vi "Code 0.0.4.vi"(8 "error in (no error)":errorcluster, 9 "Drv":u8(ring) items=["Drv 1", "Drv 2"], 10 "Port":u16=8030) -> (0 "error out":errorcluster)   [LabVIEW 2017]
panel:
  out "Array 2":u8[][](array[numeric])
  out "Array":u16[](array[numeric])
  in  "x":bool
  out "array":i32[][](array[numeric])
  out "O":i32[](array[numeric])
  out "Data1Send":bool
  out "DataBSend":bool
  out "Array 5":u16[](array[numeric]) format="%.0x"
  out "Array 4":u16[](array[numeric]) format="%.0x"
  out "Numeric":i32
  out "CheckSumData2":u16 format="%.0x"
  in  "DataBSendFlag":bool
  out "CheckSumData1":u16 format="%.0x"
  in  "Data1SendFlag":bool
  in  "HeaderFlag":bool
  out "(hi.lo) 3":u16 format="%.0x"
  out "(hi.lo) 2":u16 format="%.0x"
  out "Drv Out":u8[](array[numeric]) format="%.0x"
  out "E1b":u8 format="%.0x"
  in  "CatchNetworkFlag":bool
  out "E1a":u8 format="%.0x"
  out "State":i32
  in  "stop Listen":bool
  in  "status":bool
  out "conn ID":refnum<k5>
  out "Error List":string
  in  "Next Button":bool
  in  "File Path Control":path
  out "Status":bool
  out "cmd Sent":bool
  out "CheckSumArray":u16[][](array[numeric]) format="%.0x"
  out "CheckSum":bool[][](array[boolean])
  out "CheckSum DataB":u16 format="%.0x"
  out "CheckSum Data":u16 format="%.0x"
  out "Array 3":u16[][](array[numeric]) format="%.0x"
  out "Num of Data packet":i32
  out "Writting Data":bool
  out "Size of Text File":i32
  out "Full Text File":u8[](array[numeric]) format="%.0x"
  out "All bytes in file in HEX U8":u8[](array[numeric]) format="%02x"
  out "Send Header":bool
  out "AutoBaud Success":bool
  out "sumHeader":u16 format="%.0x"
  in  "AutoBaudFalg":bool
  # "Ver 0.0.4"
  # "Header"
  # "AA08 0000 0000 0000 0000 0000 0000 0000 0000 3E00 8DE6"
  # "Boot\n495D 4100 0001 0000 0050 F8"
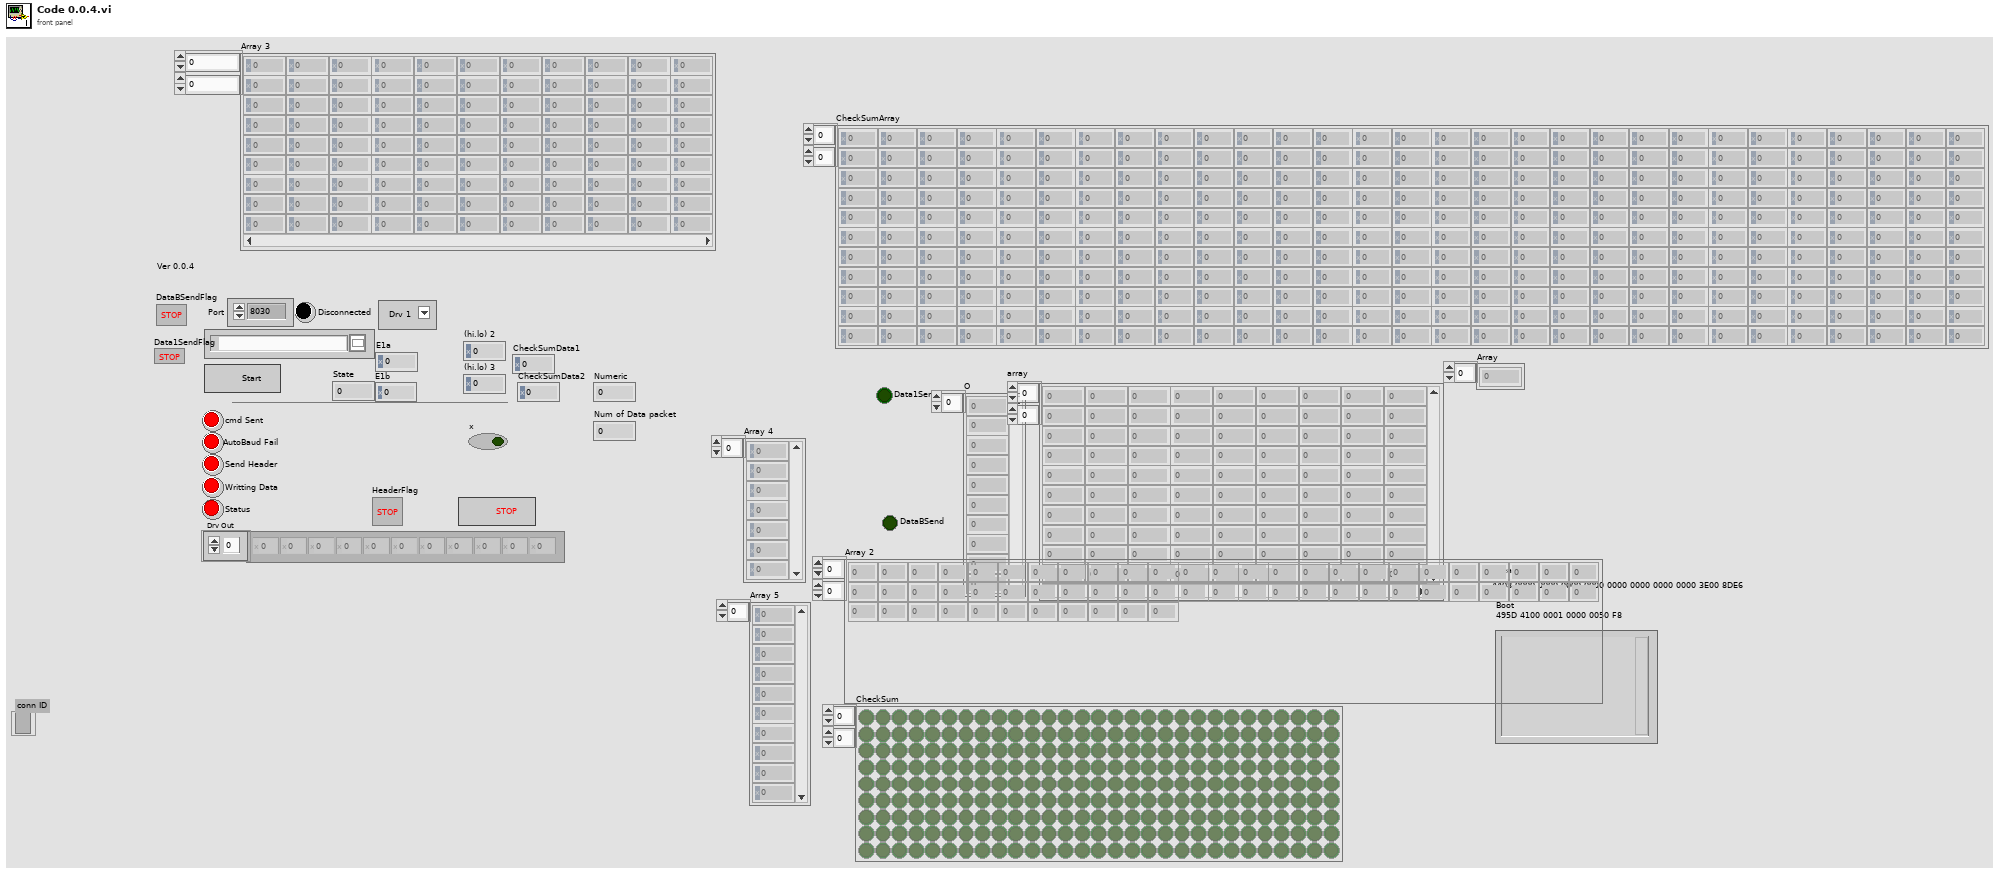
[diagram p1: front panel]
types:
  T1 = enum16{"open", "replace", "create", "open or create", "replace or create", "replace or create with confirmation"}
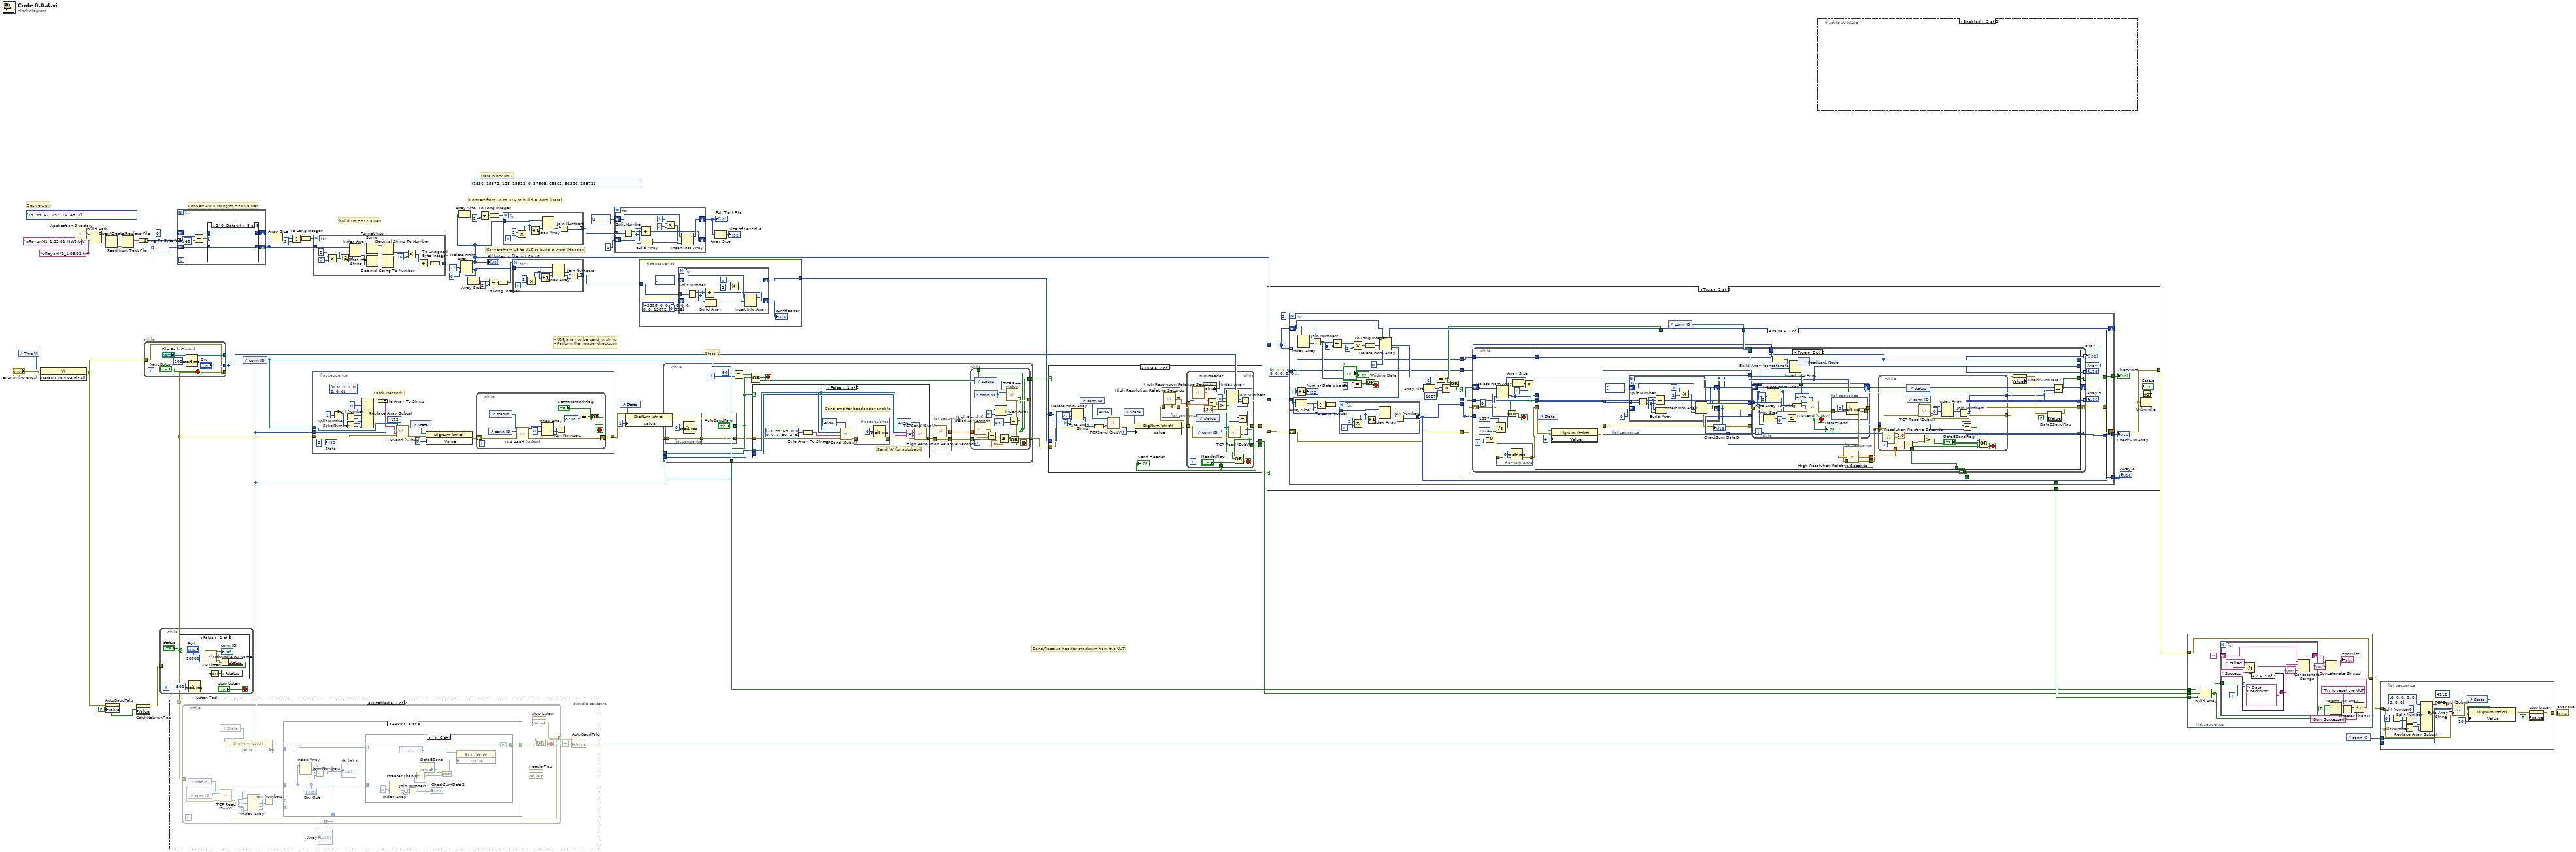
[diagram p0: block diagram]
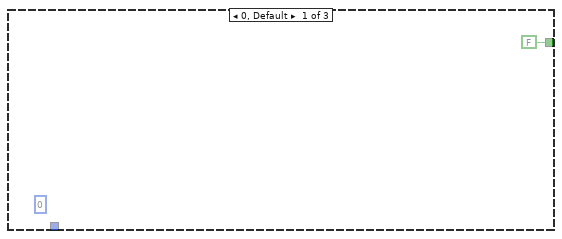
[diagram p2: hidden frame]
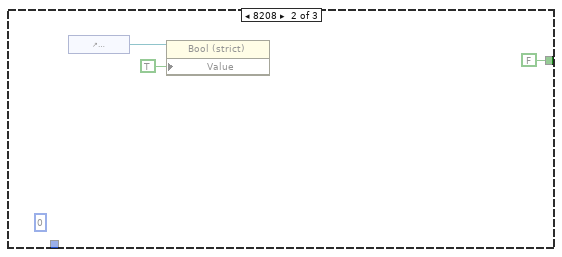
[diagram p3: hidden frame]
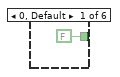
[diagram p4: hidden frame]
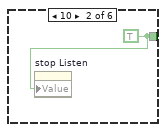
[diagram p5: hidden frame]
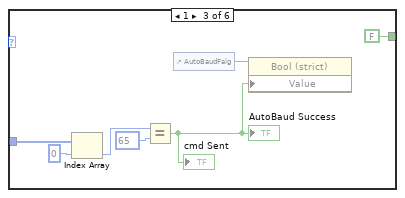
[diagram p6: hidden frame]
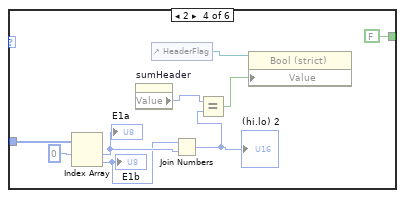
[diagram p7: hidden frame]
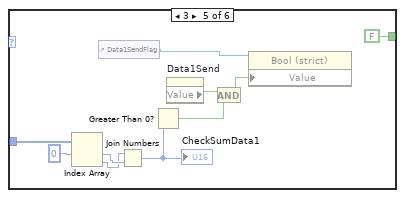
[diagram p8: hidden frame]
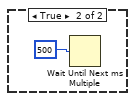
[diagram p11: hidden frame]
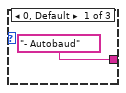
[diagram p12: hidden frame]
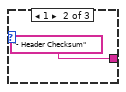
[diagram p13: hidden frame]
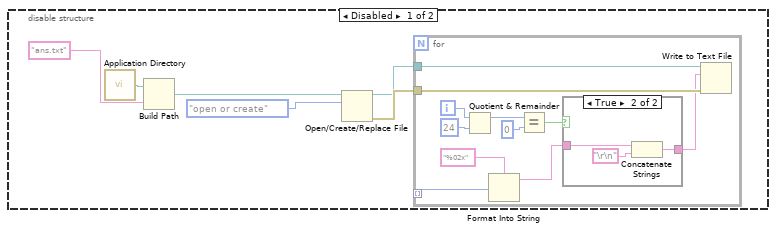
[diagram p14: hidden frame]
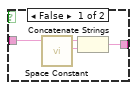
[diagram p15: hidden frame]
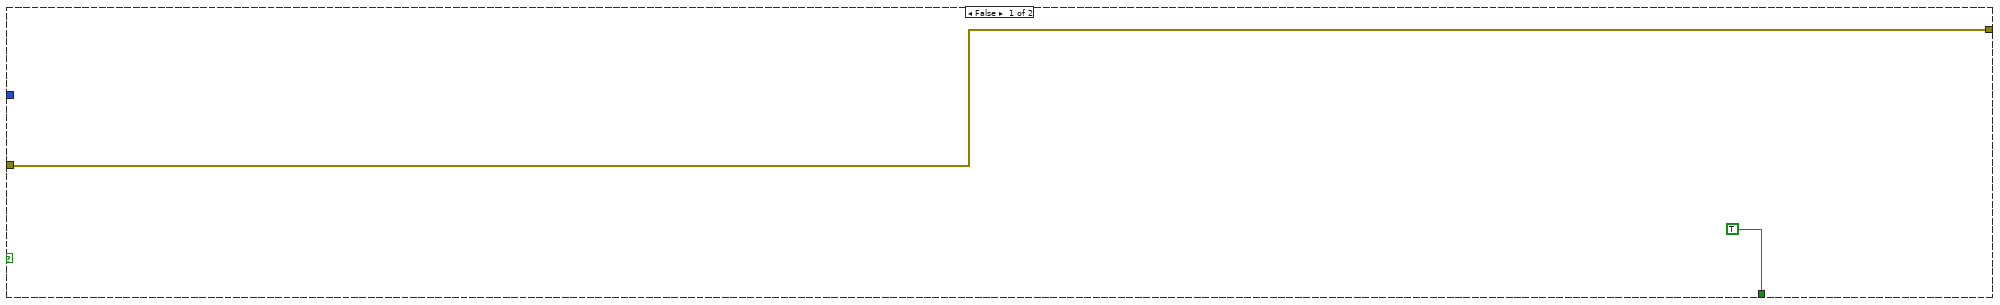
[diagram p16: hidden frame]
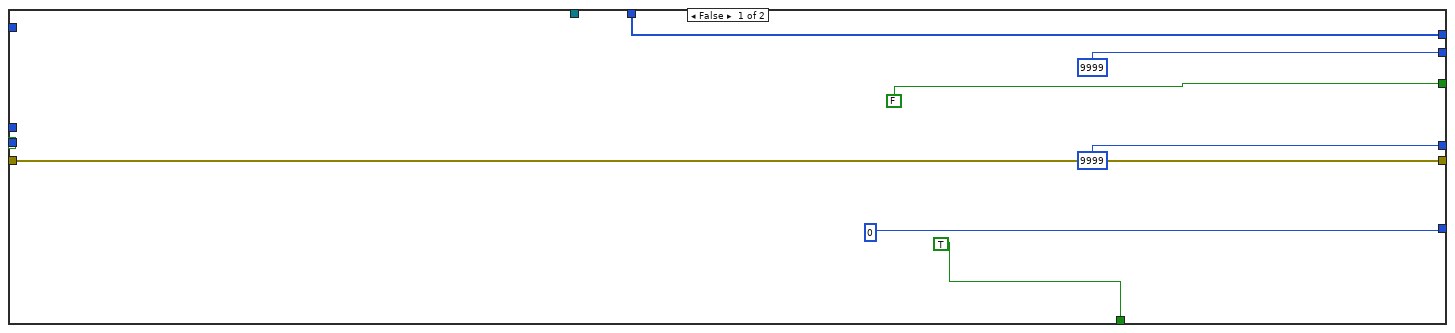
[diagram p17: hidden frame]
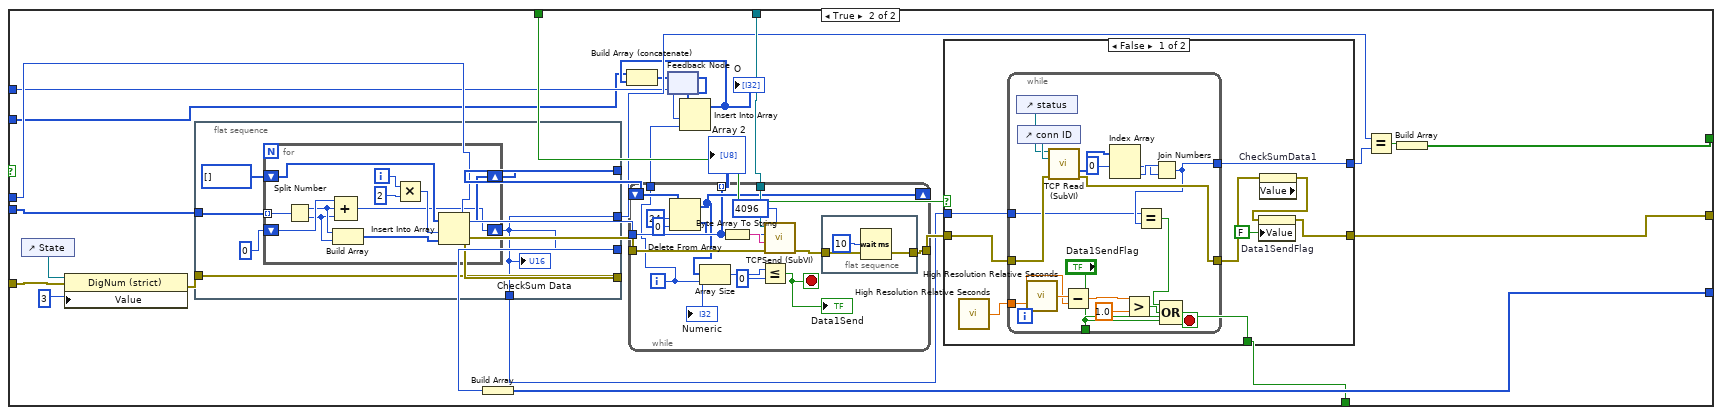
[diagram p18: hidden frame]
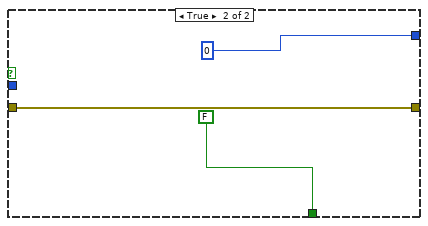
[diagram p19: hidden frame]
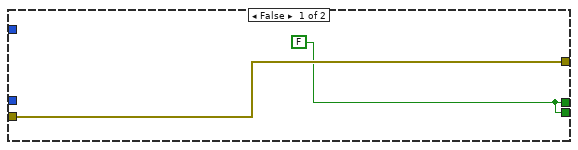
[diagram p20: hidden frame]
diagram:
  (unwired) u8[] [73, 93, 62, 192, 16, 48, 0] ("output array")
  w13 = FALSE ("stop")
  (unwired) u16[] [1536, 15872, 128, 15912, 0, 37503, 63861, 36326, 15872] ("Array 4")
  (unwired) "uRayonM1_1.05.01_HW2.txt" ("name or relative path")
  # "Data Block No 1"
  # "Get version"
  # "State 1"
  # "Send/Receive header checksum from the UUT"
  # "- U16 array to be send in string\n- Perform the header checksum"
  # "Convert from U8 to U16 to build a word (Header)"
  # "build U8 HEX values"
  # "Convert from U8 to U16 to build a word (Data)"
  # "Convert ASCII string to HEX values"
  n1 = control-ref of="This VI"() -> (w27:refnum<vi>)
  n2 = invoke class="VI" method="Default Vals.Reinit All"(reference=w27, error in="error in (no error)") -> (error out=w15:errorcluster)  [unwired: 1 in, 2 out]
  n3 = call <vilib>:"Application Directory.vi"() -> ("Application Directory"=w58:path)
  n4 = Build Path(base path=w58, name or relative path="uRayonM1_1.03.02.txt") -> (appended path=w25:path)
  n5 = property on="AutoBaudFalg" class="Bool (strict)"(error in=w15, "Value"=w13) -> (error out=w12:errorcluster)  [unwired: 1 in, 1 out]
  n6 = Open/Create/Replace File(file path (use dialog)=w25) -> (refnum out=w56:refnum<file>, error out=w57:errorcluster)  [unwired: 5 in, 1 out]
  n7 = Read from Text File(file (use dialog)=w56, error in=w57) -> (text=w54:string)  [unwired: 2 in, 3 out]
  n8 = property on="CatchNetworkFlag" class="Bool (strict)"(error in=w12, "Value"=w13) -> (error out=w11:errorcluster)  [unwired: 1 in, 1 out]
  n9 = String To Byte Array(string=w54) -> (unsigned byte array=w55:u8[])
  n10 = while {
    tunnel: ["File Path Control"] -> _
    tunnel: w15 -> [w59]
    tunnel: ["Drv"] -> w23
    tunnel: [w59] -> w3
    stop <- "Next Button" stop-if-true
    n11 = Wait (ms)(milliseconds to wait=u32 200) -> ()  [unwired: 1 out]
  }
  n12 = while "Listen Task" {
    tunnel: w11 -> [_]
    stop <- "stop Listen" stop-if-true
    n13 = case shown="False" "status" {
      frame False {
        n14 = call <vilib>:"TCP Listen.vi"("timeout ms (wait forever: -1)"=10000, "port"="Port") -> ("error out"=w70:errorcluster, "connection ID"=→"conn ID":refnum<k5>)  [unwired: 5 in, 3 out]
        n15 = Unbundle By Name(w70) -> ("status"=w67:bool)
        n16 = Not(x=w67) -> (.not. x?=w68:bool)
        n17 = local write "status"(w68) -> ()
      }
      frame True {
        n18 = Wait Until Next ms Multiple(millisecond multiple=u32 500) -> ()  [unwired: 1 out]
      }
    }
    n19 = Wait (ms)(milliseconds to wait=u32 500) -> ()  [unwired: 1 out]
  }
  n20 = disable-structure shown="Disabled" {
    disable-tunnel: w3 -> [w75 _]
    frame Disabled {
      n21 = while {
        tunnel: [w80] -> w76
        tunnel: w75 -> [w79]
        tunnel: [w78] -> w74 mode=indexing
        stop <- w94 stop-if-true
        n22 = control-ref of="status"() -> (w91:refnum<vi>)
        n23 = control-ref of="conn ID"() -> (w92:refnum<vi>)
        n24 = control-ref of="State"() -> (w82:refnum<vi>)
        n25 = call "TCP Read (SubVI).vi"("Status in"=w91, "TCP in"=w92, "error in (no error)"=w79) -> ("Rx data tmp"=w90:u8[], "Drv Array"=w89:u8[], "error out"=w80:errorcluster)  [unwired: 2 in, 8 out]
        n26 = property class="DigNum (strict)"(reference=w82) -> ("Value"=w81:i32)  [unwired: 1 in, 2 out]
        n27 = Index Array(array=w90, index #1=0 ("index"), index #3=4 ("index")) -> (element #1=w87:u8, element #2=w88:u8, element #3=w83:u8)  [unwired: 1 in]
        n28 = Join Numbers(hi=w88, lo=w87) -> ((hi.lo)=w85:u16)
        n29 = case shown="2000" w85 {
          tunnel: w89 -> [_ _ w104]
          tunnel: [FALSE FALSE w105] -> w95
          tunnel: w83 -> [_ _ _]
          tunnel: w81 -> [_ _ w101]
          tunnel: [_ _ w100] -> w78
          frame 0, Default {
            (unwired) u16 0
          }
          frame 8208 {
            (unwired) u16 0
            n30 = control-ref of="CatchNetworkFlag"() -> (w99:refnum<vi>)
            n31 = property class="Bool (strict)"(reference=w99, "Value"=TRUE) -> ()  [unwired: 1 in, 2 out]
          }
          frame 8192 {
            n32 = Index Array(array=w104) -> (element #1=w102:u8, element #2=w103:u8)  [unwired: 2 in]
            n33 = Join Numbers(hi=w103, lo=w102) -> ((hi.lo)=w100:u16)
            "(hi.lo) 3" <- w100
            n34 = case shown="4" w101 {
              tunnel: w104 -> [_ _ w113 w123 w133 w143]
              tunnel: [FALSE w107 FALSE FALSE FALSE FALSE] -> w105
              frame 0, Default {
              }
              frame 10 {
                w107 = TRUE
                n35 = property on="stop Listen" class="Bool (strict)"("Value"=w107) -> ()  [unwired: 2 in, 2 out]
              }
              frame 1 {
                n36 = Index Array(array=w113, index=0) -> (element=w110:u8)
                n37 = Equal?(x=w110, y=u8 65) -> (x = y?=w108:bool)
                "AutoBaud Success" <- w108
                "cmd Sent" <- w108
                n38 = control-ref of="AutoBaudFalg"() -> (w114:refnum<vi>)
                n39 = property class="Bool (strict)"(reference=w114, "Value"=w108) -> ()  [unwired: 1 in, 2 out]
              }
              frame 2 {
                n40 = Index Array(array=w123, index #1=0 ("index")) -> (element #1=w120:u8, element #2=w119:u8)  [unwired: 1 in]
                "E1a" <- w120
                "E1b" <- w119
                n41 = property on="sumHeader" class="DigNum (strict)"() -> ("Value"=w115:u16)  [unwired: 2 in, 2 out]
                n42 = control-ref of="HeaderFlag"() -> (w118:refnum<vi>)
                n43 = Join Numbers(hi=w119, lo=w120) -> ((hi.lo)=w116:u16)
                "(hi.lo) 2" <- w116
                n44 = Equal?(x=w115, y=w116) -> (x = y?=w117:bool)
                n45 = property class="Bool (strict)"(reference=w118, "Value"=w117) -> ()  [unwired: 1 in, 2 out]
              }
              frame 3 {
                n46 = Index Array(array=w133, index #1=0 ("index")) -> (element #1=w130:u8, element #2=w127:u8)  [unwired: 1 in]
                n47 = control-ref of="Data1SendFlag"() -> (w128:refnum<vi>)
                n48 = Join Numbers(hi=w127, lo=w130) -> ((hi.lo)=w126:u16)
                "CheckSumData1" <- w126
                n49 = Greater Than 0?(x=w126) -> (x > 0?=w129:bool)
                n50 = property on="Data1Send" class="Bool (strict)"() -> ("Value"=w124:bool)  [unwired: 2 in, 2 out]
                n51 = And(x=w124, y=w129) -> (x .and. y?=w125:bool)
                n52 = property class="Bool (strict)"(reference=w128, "Value"=w125) -> ()  [unwired: 1 in, 2 out]
              }
              frame 4 {
                n53 = Index Array(array=w143, index #1=0 ("index")) -> (element #1=w140:u8, element #2=w137:u8)  [unwired: 1 in]
                n54 = control-ref of="DataBSendFlag"() -> (w138:refnum<vi>)
                n55 = Join Numbers(hi=w137, lo=w140) -> ((hi.lo)=w136:u16)
                "CheckSumData2" <- w136
                n56 = Greater Than 0?(x=w136) -> (x > 0?=w139:bool)
                n57 = property on="DataBSend" class="Bool (strict)"() -> ("Value"=w134:bool)  [unwired: 2 in, 2 out]
                n58 = And(x=w134, y=w139) -> (x .and. y?=w135:bool)
                n59 = property class="Bool (strict)"(reference=w138, "Value"=w135) -> ()  [unwired: 1 in, 2 out]
              }
            }
            "Drv Out" <- w104
          }
        }
        n60 = property on="HeaderFlag" class="Bool (strict)" props=["Value"]() -> ()  [unwired: 2 in, 3 out]
        n61 = property on="stop Listen" class="Bool (strict)"() -> ("Value"=w93:bool)  [unwired: 2 in, 2 out]
        n62 = Compound Arithmetic op=OR(w93, w95) -> (w94:bool)
      }
      "Array" <- w74
      n63 = property on="AutoBaudFalg" class="Bool (strict)"(error in=w76, "Value"=TRUE ("stop")) -> ()  [unwired: 1 in, 2 out]
    }
    frame Enabled {
    }
  }
  n64 = for {
    tunnel: w55 -> [w150] mode=indexing
    shift-right: [w146] -> w51
    shift-left: u8[] [] -> [w147]
    shift-right: [w145] -> _
    shift-left: 0 ("y") -> [w144]
    n65 = Subtract(x=w150, y=u8 48) -> (x-y=w148:u8)
    n66 = case shown="240, Default" w148 {
      selector: w148 -> [_ _ _ _ _ _ w184 _]
      tunnel: [w153 w158 w164 w168 w173 w178 w183 w187] -> w146
      tunnel: w147 -> [w155 w159 w165 w170 w175 w180 w185 w187]
      tunnel: [w151 w156 w161 w166 w171 w176 w181 w186] -> w145
      tunnel: w144 -> [w152 w157 w162 w167 w172 w177 w182 w186]
      frame 17, 49 {
        n67 = Increment(x=w152) -> (x+1=w151:i32)
        n68 = Insert Into Array(array=w155, index=w152, new element=u8 10) -> (w153:u8[])
      }
      frame 18, 50 {
        n69 = Increment(x=w157) -> (x+1=w156:i32)
        n70 = Insert Into Array(array=w159, index=w157, new element=u8 11) -> (w158:u8[])
      }
      frame 19, 51 {
        n71 = Increment(x=w162) -> (x+1=w161:i32)
        n72 = Insert Into Array(array=w165, index=w162, new element=u8 12) -> (w164:u8[])
      }
      frame 20, 52 {
        n73 = Increment(x=w167) -> (x+1=w166:i32)
        n74 = Insert Into Array(array=w170, index=w167, new element=u8 13) -> (w168:u8[])
      }
      frame 21, 53 {
        n75 = Increment(x=w172) -> (x+1=w171:i32)
        n76 = Insert Into Array(array=w175, index=w172, new element=u8 14) -> (w173:u8[])
      }
      frame 22, 54 {
        n77 = Increment(x=w177) -> (x+1=w176:i32)
        n78 = Insert Into Array(array=w180, index=w177, new element=u8 15) -> (w178:u8[])
      }
      frame 0..9 {
        n79 = Insert Into Array(array=w185, index=w182, new element=w184) -> (w183:u8[])
        n80 = Increment(x=w182) -> (x+1=w181:i32)
      }
      frame 240, Default {
      }
    }
  }
  n81 = control-ref of="conn ID"() -> (w5:refnum<vi>)
  n82 = Array Size(array=w51) -> (size(s)=w50:i32)
  n83 = Divide(x=w50, y=2) -> (x/y=w48:dbl)
  n84 = To Long Integer(number=w48) -> (32bit integer=w47:i32)
  n85 = flat-sequence {
    tunnel: w3 -> [w207]
    tunnel: w5 -> [w206]
    tunnel: w23 -> [w205]
    tunnel: [w193] -> w22
    frame #0 {
      # "Catch Network"
      n86 = Split Number(x=u32 1) -> (hi(x)=w203:u16, lo(x)=w202:u16)
      n87 = Split Number(x=w202) -> (hi(x)=w197:u8, lo(x)=w196:u8)
      n88 = Split Number(x=w203) -> (hi(x)=w195:u8, lo(x)=w194:u8)
      n89 = Replace Array Subset(array=u8[] [0, 0, 0, 0, 0, 0, 0, 0] ("unsigned byte array"), new element #1=w196, index #1=0 ("index"), new element #2=w197, new element #3=w194, new element #4=w195) -> (w198:u8[])  [unwired: 3 in]
      n90 = Byte Array To String(unsigned byte array=w198) -> (string=w204:string)
      n91 = call "TCPSend (SubVI).vi"("Opcode"=u32 4112, "error in"=w207, "string"=w204, "Drv"=w205, "RefNum in"=w206) -> ("error out"=w191:errorcluster)  [unwired: 6 in]
      n92 = control-ref of="State"() -> (w192:refnum<vi>)
      n93 = property class="DigNum (strict)"(reference=w192, error in=w191, "Value"=0) -> (error out=w188:errorcluster)  [unwired: 1 out]
      n94 = while {
        shift-right: [w220] -> w193
        shift-left: w188 -> [w221]
        stop <- w215 stop-if-true
        n95 = control-ref of="conn ID"() -> (w213:refnum<vi>)
        n96 = control-ref of="status"() -> (w214:refnum<vi>)
        n97 = call "TCP Read (SubVI).vi"("Status in"=w214, "TCP in"=w213, "error in (no error)"=w221) -> ("Rx data tmp"=w212:u8[], "error out"=w220:errorcluster)  [unwired: 2 in, 9 out]
        n98 = Index Array(array=w212, index #1=0 ("index")) -> (element #1=w211:u8, element #2=w210:u8)  [unwired: 1 in]
        n99 = Join Numbers(hi=w210, lo=w211) -> ((hi.lo)=w219:u16)
        n100 = Equal?(x=w219, y=u16 8208) -> (x = y?=w217:bool)
        n101 = Or(x="CatchNetworkFlag", y=w217) -> (x .or. y?=w215:bool)
      }
      "State" <- 0 ("State")
    }
  }
  n102 = for {
    N: w47 -> [_]
    tunnel: w51 -> [w236]
    tunnel: [w222] -> w46 mode=indexing
    i -> [w235]
    n103 = Multiply(x=2, y=w235) -> (x*y=w233:i32)
    n104 = Increment(x=w233) -> (x+1=w232:i32)
    n105 = Index Array(array=w236, index #1=w233, index #2=w232) -> (element #1=w225:u8, element #2=w224:u8)
    n106 = Format Into String(w225) -> (resulting string=w226:string)  [unwired: 3 in, 1 out]
    n107 = Format Into String(w224) -> (resulting string=w231:string)  [unwired: 3 in, 1 out]
    n108 = Decimal String To Number(string=w226) -> (number=w227:i32)  [unwired: 2 in, 1 out]
    n109 = Decimal String To Number(string=w231) -> (number=w230:i32)  [unwired: 2 in, 1 out]
    n110 = Multiply(x=w227, y=16) -> (x*y=w229:i32)
    n111 = Add(x=w229, y=w230) -> (x+y=w223:i32)
    n112 = To Unsigned Byte Integer(number=w223) -> (unsigned 8bit integer=w222:u8)
  }
  n113 = Delete From Array(array=w46, length=22, index=0) -> (deleted portion=w35:u8[], array with subset deleted=w28:u8[])
  "All bytes in file in HEX U8" <- w28
  n114 = Array Size(array=w28) -> (size(s)=w41:i32)
  n115 = Array Size(array=w35) -> (size(s)=w40:i32)
  n116 = Divide(x=w41, y=2) -> (x/y=w43:dbl)
  n117 = Divide(x=w40, y=2) -> (x/y=w38:dbl)
  n118 = To Long Integer(number=w43) -> (32bit integer=w36:i32)
  n119 = To Long Integer(number=w38) -> (32bit integer=w37:i32)
  n120 = for {
    N: w36 -> [_]
    tunnel: w28 -> [w241]
    tunnel: [w237] -> w29 mode=indexing
    i -> [w240]
    n121 = Multiply(x=2, y=w240) -> (x*y=w243:i32)
    n122 = Increment(x=w243) -> (x+1=w244:i32)
    n123 = Index Array(array=w241, index #1=w243, index #2=w244) -> (element #1=w239:u8, element #2=w238:u8)
    n124 = Join Numbers(hi=w239, lo=w238) -> ((hi.lo)=w237:u16)
  }
  n125 = for {
    N: w37 -> [_]
    tunnel: w35 -> [w249]
    tunnel: [w245] -> w34 mode=indexing
    i -> [w248]
    n126 = Multiply(x=2, y=w248) -> (x*y=w251:i32)
    n127 = Increment(x=w251) -> (x+1=w252:i32)
    n128 = Index Array(array=w249, index #1=w251, index #2=w252) -> (element #1=w247:u8, element #2=w246:u8)
    n129 = Join Numbers(hi=w247, lo=w246) -> ((hi.lo)=w245:u16)
  }
  n130 = for {
    tunnel: w29 -> [w263] mode=indexing
    shift-right: [w258] -> w31
    shift-left: u8[] [] -> [w257]
    shift-right: [w255] -> _
    shift-left: u16 0 -> [w256]
    i -> [w262]
    n131 = Split Number(x=w263) -> (hi(x)=w254:u8, lo(x)=w253:u8)
    n132 = Build Array(w254, w253) -> (w260:u8[])
    n133 = Compound Arithmetic op=ADD(w256, w254, w253) -> (w255:u16)
    n134 = Multiply(x=w262, y=2) -> (x*y=w259:i32)
    n135 = Insert Into Array(array=w257, index=w259, new element=w260) -> (w258:u8[])
  }
  "Full Text File" <- w31
  n136 = control-ref of="State"() -> (w18:refnum<vi>)
  n137 = property class="DigNum (strict)"(reference=w18, error in=w22, "Value"=1) -> (error out=w16:errorcluster)  [unwired: 1 out]
  n138 = flat-sequence {
    tunnel: [w266] -> w19
    tunnel: w34 -> [w265]
    frame #0 {
      (unwired) u16[] [43528, 0, 0, 0, 0, 0, 0, 0, 0, 15872, 36326]
      n139 = for {
        tunnel: w265 -> [w279] mode=indexing
        shift-right: [w274] -> w266
        shift-left: u8[] [] -> [w273]
        shift-right: [w271] -> w264
        shift-left: u16 0 -> [w272]
        i -> [w278]
        n140 = Split Number(x=w279) -> (hi(x)=w270:u8, lo(x)=w269:u8)
        n141 = Build Array(w270, w269) -> (w276:u8[])
        n142 = Compound Arithmetic op=ADD(w272, w270, w269) -> (w271:u16)
        n143 = Multiply(x=w278, y=2) -> (x*y=w275:i32)
        n144 = Insert Into Array(array=w273, index=w275, new element=w276) -> (w274:u8[])
      }
      "sumHeader" <- w264
    }
  }
  n145 = while {
    tunnel: w16 -> [w293]
    tunnel: [w281] -> w10
    tunnel: w23 -> [w295]
    tunnel: w5 -> [w294]
    tunnel: [w287] -> w9
    tunnel: [w280] -> w2
    i -> [w290]
    stop <- w292 stop-if-true
    n146 = flat-sequence {
      tunnel: w293 -> [w314]
      tunnel: [w314] -> w288
      tunnel: [w316] -> w284
      tunnel: w288 -> [w316]
      tunnel: ["AutoBaudFalg"] -> w287
      frame #0 {
        n147 = Wait (ms)(milliseconds to wait=u32 0) -> ()  [unwired: 1 out]
      }
      frame #1 {
      }
    }
    n148 = Equal?(x=90, y=w290) -> (x = y?=w291:bool)
    n149 = case shown="False" w287 {
      tunnel: w284 -> [w327 w330]
      tunnel: w295 -> [w326 _]
      tunnel: w294 -> [w325 _]
      tunnel: [w318 w330] -> w282
      frame False {
        # "Send 'A' for autobaud"
        # "Send cmd for bootloader enable"
        n150 = Byte Array To String(unsigned byte array=u8[] [73, 93, 65, 0, 0, 1, 0, 0, 0, 80, 248] ("output array")) -> (string=w321:string)
        n151 = call "TCPSend (SubVI).vi"("Opcode"=u32 4096, "error in"=w327, "string"=w321, "Drv"=w326, "RefNum in"=w325) -> ("error out"=w323:errorcluster)  [unwired: 6 in]
        n152 = flat-sequence {
          tunnel: w323 -> [w328]
          tunnel: [w328] -> w322
          frame #0 {
            n153 = Wait (ms)(milliseconds to wait=u32 0) -> ()  [unwired: 1 out]
          }
        }
        n154 = call "TCPSend (SubVI).vi"("Opcode"=u32 4096, "error in"=w322, "string"="A" ("write buffer"), "Drv"=w326, "RefNum in"=w325) -> ("error out"=w318:errorcluster)  [unwired: 6 in]
      }
      frame True {
      }
    }
    n155 = flat-sequence {
      tunnel: w282 -> [w297]
      tunnel: [w297] -> w286
      tunnel: [w296] -> w285
      frame #0 {
        n156 = call <vilib>:"High Resolution Relative Seconds.vi"() -> ("relative seconds"=w296:dbl)
      }
    }
    n157 = while {
      tunnel: w286 -> [w301]
      tunnel: w285 -> [w307]
      tunnel: [w300] -> w281
      tunnel: [w298] -> w283
      tunnel: [w298] -> w280
      stop <- w299 stop-if-true
      n158 = control-ref of="status"() -> (w311:refnum<vi>)
      n159 = control-ref of="conn ID"() -> (w312:refnum<vi>)
      n160 = call <vilib>:"High Resolution Relative Seconds.vi"() -> ("relative seconds"=w308:dbl)
      n161 = Subtract(x=w308, y=w307) -> (x-y=w306:dbl)
      n162 = Greater Or Equal?(x=w306, y=2.0) -> (x >= y?=w304:bool)
      n163 = call "TCP Read (SubVI).vi"("Status in"=w311, "TCP in"=w312, "error in (no error)"=w301) -> ("Drv Array"=w309:u8[], "error out"=w300:errorcluster)  [unwired: 2 in, 9 out]
      n164 = Index Array(array=w309, index=0) -> (element=w303:u8)
      n165 = Equal?(x=w303, y=u8 65) -> (x = y?=w298:bool)
      n166 = Or(x=w298, y=w304) -> (x .or. y?=w299:bool)
    }
    n167 = Compound Arithmetic op=OR(w291, w287, w283) -> (w292:bool)
  }
  n168 = Array Size(array=w31) -> (size(s)=→"Size of Text File":i32)
  n169 = case shown="True" w2 {
    tunnel: w10 -> [w332 w348]
    tunnel: [w332 w350] -> w20
    tunnel: w19 -> [_ w349]
    tunnel: [w331 w337] -> w8
    tunnel: w23 -> [_ w347]
    tunnel: [w331 w333] -> w1
    frame False {
      w331 = FALSE
    }
    frame True {
      n170 = Delete From Array(array=w349, length=22, index=0) -> (deleted portion=w341:u8[])  [unwired: 1 out]
      n171 = control-ref of="conn ID"() -> (w338:refnum<vi>)
      n172 = Byte Array To String(unsigned byte array=w341) -> (string=w339:string)
      n173 = call "TCPSend (SubVI).vi"("Opcode"=u32 4096, "error in"=w348, "string"=w339, "Drv"=w347, "RefNum in"=w338) -> ("error out"=w344:errorcluster)  [unwired: 6 in]
      n174 = control-ref of="State"() -> (w346:refnum<vi>)
      n175 = property class="DigNum (strict)"(reference=w346, error in=w344, "Value"=2) -> (error out=w336:errorcluster)  [unwired: 1 out]
      n176 = flat-sequence {
        tunnel: w336 -> [w351]
        tunnel: [w351] -> _
        tunnel: [w352] -> w334
        tunnel: [w351] -> w335
        frame #0 {
          n177 = call <vilib>:"High Resolution Relative Seconds.vi"() -> ("relative seconds"=w352:dbl)
        }
      }
      n178 = while {
        tunnel: w335 -> [w363]
        tunnel: [w362] -> w350
        tunnel: ["HeaderFlag"] -> w337
        tunnel: w334 -> [w368]
        tunnel: [w353] -> w333
        stop <- w359 stop-if-true
        n179 = call <vilib>:"High Resolution Relative Seconds.vi"() -> ("relative seconds"=w369:dbl)
        n180 = control-ref of="status"() -> (w365:refnum<vi>)
        n181 = control-ref of="conn ID"() -> (w364:refnum<vi>)
        n182 = property on="sumHeader" class="DigNum (strict)"() -> ("Value"=w354:u16)  [unwired: 2 in, 2 out]
        n183 = Subtract(x=w369, y=w368) -> (x-y=w367:dbl)
        n184 = Greater Or Equal?(x=w367, y=15.0) -> (x >= y?=w358:bool)
        n185 = call "TCP Read (SubVI).vi"("Status in"=w365, "TCP in"=w364, "error in (no error)"=w363) -> ("Drv Array"=w360:u8[], "error out"=w362:errorcluster)  [unwired: 2 in, 9 out]
        n186 = Index Array(array=w360, index #1=0 ("index")) -> (element #1=w356:u8, element #2=w357:u8)  [unwired: 1 in]
        n187 = Join Numbers(hi=w357, lo=w356) -> ((hi.lo)=w355:u16)
        n188 = Equal?(x=w355, y=w354) -> (x = y?=w353:bool)
        n189 = Compound Arithmetic op=OR(w353, w358, "HeaderFlag") -> (w359:bool)
      }
      "Send Header" <- w337
    }
  }
  n190 = case shown="True" w1 {
    tunnel: w20 -> [w372 w380]
    tunnel: [w372 w379] -> w14
    tunnel: w28 -> [_ w383]
    tunnel: [TRUE w376] -> w24
    tunnel: w23 -> [_ w375]
    frame False {
    }
    frame True {
      n191 = for {
        N: 3 -> [_]
        shift-right: [w411] -> _
        shift-left: w383 -> [w421]
        tunnel: w383 -> [_] mode=indexing
        tunnel: [w404] -> w384 mode=indexing
        tunnel: [w400] -> w382 mode=indexing
        tunnel: [w399] -> w381 mode=indexing
        shift-right: [w389] -> w379
        shift-left: w380 -> [w393]
        tunnel: [w392] -> w376
        tunnel: w375 -> [w391]
        tunnel: i32[] [0, 0, 0, 0, 0, 0, 0, 0, 0, 0, 0] ("array") -> [w387]
        i -> [w388]
        stop <- w386 stop-if-true
        n192 = Increment(x=w388) -> (x+1=→"Num of Data packet":i32)
        n193 = Index Array(array=w421) -> (element #1=w420:u8, element #2=w419:u8)  [unwired: 2 in]
        n194 = Join Numbers(hi=w419, lo=w420) -> ((hi.lo)=w395:u16)
        n195 = Add(x=w395, y=u32 3) -> (x+y=w417:u32)
        n196 = Equal?(x=w395, y=u16 0) -> (x = y?=w414:bool)
        "Writting Data" <- w414
        n197 = Multiply(x=w417, y=u32 2) -> (x*y=w415:u32)
        n198 = To Long Integer(number=w415) -> (32bit integer=w396:i32)
        n199 = Or(x="x", y=w414) -> (x .or. y?=w386:bool)
        n200 = Delete From Array(array=w421, length=w396, index=0) -> (deleted portion=w397:u8[], array with subset deleted=w411:u8[])
        n201 = Array Size(array=w397) -> (size(s)=w408:i32)
        n202 = Divide(x=w408, y=2) -> (x/y=w410:dbl)
        n203 = To Long Integer(number=w410) -> (32bit integer=w407:i32)
        n204 = for {
          N: w407 -> [_]
          tunnel: w397 -> [w649]
          tunnel: [w645] -> w404 mode=indexing
          i -> [w648]
          n205 = Multiply(x=2, y=w648) -> (x*y=w651:i32)
          n206 = Increment(x=w651) -> (x+1=w652:i32)
          n207 = Index Array(array=w649, index #1=w651, index #2=w652) -> (element #1=w647:u8, element #2=w646:u8)
          n208 = Join Numbers(hi=w647, lo=w646) -> ((hi.lo)=w645:u16)
        }
        n209 = Array Size(array=w404) -> (size(s)=w406:i32)
        n210 = Equal?(x=w396, y=6) -> (x = y?=w394:bool)
        n211 = Less Or Equal?(x=w406, y=1027) -> (x <= y?=w402:bool)
        n212 = Or(x=w394, y=w402) -> (x .or. y?=w401:bool)
        n213 = control-ref of="conn ID"() -> (w390:refnum<vi>)
        n214 = case shown="False" w401 {
          tunnel: w393 -> [w433 w561]
          tunnel: [w434 w579] -> w389
          tunnel: w404 -> [w431 w578]
          tunnel: [w432 w575] -> w400
          tunnel: [w430 w573] -> w399
          tunnel: w394 -> [_ w572]
          tunnel: [w429 w571] -> w392
          tunnel: w391 -> [w428 w567]
          tunnel: w390 -> [w427 w568]
          tunnel: w388 -> [w424 w559]
          tunnel: w387 -> [w423 w557]
          frame False {
            n215 = while {
              tunnel: w431 -> [_]
              tunnel: [w459] -> w432 mode=indexing
              shift-right: [w460] -> w434
              shift-left: w433 -> [w436]
              shift-right: [w451] -> _
              shift-left: w431 -> [w458]
              tunnel: [w450] -> w430 mode=indexing
              tunnel: [w444] -> w429
              tunnel: w428 -> [w443]
              tunnel: w427 -> [w442]
              tunnel: [w441] -> w425 mode=indexing
              tunnel: [w440] -> w426 mode=indexing
              tunnel: w424 -> [w439]
              tunnel: w423 -> [w438]
              tunnel: [w437] -> w422 mode=indexing
              i -> [w449]
              stop <- w453 stop-if-true
              n216 = Equal To 0?(x=w449) -> (x = 0?=w448:bool)
              n217 = Select(t=1027 ("length"), s=w448, f=1024 ("length")) -> (s? t:f=w445:i32)
              n218 = flat-sequence {
                tunnel: w436 -> [w461]
                tunnel: [w461] -> w435
                frame #0 {
                  n219 = Wait (ms)(milliseconds to wait=u32 0) -> ()  [unwired: 1 out]
                }
              }
              n220 = Delete From Array(array=w458, length=w445, index=0) -> (deleted portion=w452:u16[], array with subset deleted=w451:u16[])
              n221 = Array Size(array=w452) -> (size(s)=w456:i32)
              n222 = Greater?(x=w456, y=1) -> (0:w454:bool)
              n223 = Not(x=w454) -> (.not. x?=w453:bool)
              n224 = case shown="True" w454 {
                tunnel: [w469 w486] -> w460
                tunnel: w435 -> [w469 w484]
                tunnel: [FALSE w497] -> w459
                tunnel: w452 -> [_ w496]
                tunnel: [u16 0 ("Numeric") w495] -> w450
                tunnel: [TRUE w489] -> w444
                tunnel: w443 -> [_ w494]
                tunnel: w442 -> [_ w493]
                tunnel: [u16 9999 ("Value") w471] -> w441
                tunnel: [u16 9999 w482] -> w440
                tunnel: w439 -> [_ w477]
                tunnel: w438 -> [w463 w474]
                tunnel: [w463 w473] -> w437
                frame False {
                }
                frame True {
                  n225 = control-ref of="State"() -> (w492:refnum<vi>)
                  n226 = property class="DigNum (strict)"(reference=w492, error in=w484, "Value"=4) -> (error out=w485:errorcluster)  [unwired: 1 out]
                  n227 = flat-sequence {
                    tunnel: w485 -> [w537]
                    tunnel: [w539] -> w483
                    tunnel: [w536] -> w482
                    tunnel: w496 -> [w538]
                    tunnel: [w537] -> w490
                    tunnel: [w536] -> w495
                    tunnel: [w536] -> w470
                    frame #0 {
                      n228 = for {
                        tunnel: w538 -> [w552] mode=indexing
                        shift-right: [w547] -> w539
                        shift-left: u8[] [] -> [w546]
                        shift-right: [w544] -> w536
                        shift-left: u16 0 -> [w545]
                        i -> [w551]
                        n229 = Split Number(x=w552) -> (hi(x)=w543:u8, lo(x)=w542:u8)
                        n230 = Build Array(w543, w542) -> (w549:u8[])
                        n231 = Compound Arithmetic op=ADD(w545, w543, w542) -> (w544:u16)
                        n232 = Multiply(x=w551, y=2) -> (x*y=w548:i32)
                        n233 = Insert Into Array(array=w546, index=w548, new element=w549) -> (w547:u8[])
                      }
                      "CheckSum DataB" <- w536
                    }
                  }
                  n234 = while {
                    tunnel: w490 -> [w533]
                    shift-right: [w521] -> _
                    shift-left: w483 -> [w532]
                    tunnel: w494 -> [w525]
                    tunnel: w493 -> [w524]
                    tunnel: [w522] -> w480
                    tunnel: [w518] -> w478
                    i -> [w518]
                    stop <- w529 stop-if-true
                    n235 = Delete From Array(array=w532, length=24, index=0) -> (deleted portion=w519:u8[], array with subset deleted=w521:u8[])
                    n236 = Array Size(array=w521) -> (size(s)=w528:i32)
                    n237 = Less Or Equal?(x=w528, y=0) -> (x <= y?=w529:bool)
                    "DataBSend" <- w529
                    n238 = Byte Array To String(unsigned byte array=w519) -> (string=w526:string)
                    n239 = call "TCPSend (SubVI).vi"("Opcode"=u32 4096, "error in"=w533, "string"=w526, "Drv"=w525, "RefNum in"=w524) -> ("error out"=w523:errorcluster)  [unwired: 6 in]
                    n240 = flat-sequence {
                      tunnel: w523 -> [w534]
                      tunnel: [w534] -> w522
                      frame #0 {
                        n241 = Wait (ms)(milliseconds to wait=u32 0) -> ()  [unwired: 1 out]
                      }
                    }
                  }
                  n242 = feedback #1() -> (w473:i32[])  [unwired: 1 in]
                  n243 = Build Array (concatenate)(w474, w473) -> (w476:i32[])
                  n244 = Insert Into Array(array=w476, index=w477, new element=w478) -> (w475:i32[])
                  n245 = feedback-in #1(w475) -> ()
                  n246 = flat-sequence {
                    tunnel: [w499] -> w481
                    tunnel: w480 -> [w498]
                    tunnel: [w498] -> w479
                    frame #0 {
                      n247 = call <vilib>:"High Resolution Relative Seconds.vi"() -> ("relative seconds"=w499:dbl)
                    }
                  }
                  n248 = while {
                    tunnel: w479 -> [w506]
                    tunnel: ["DataBSendFlag"] -> w489
                    tunnel: w481 -> [w515]
                    tunnel: [w503] -> w472
                    tunnel: [w502] -> w471
                    tunnel: w470 -> [w501]
                    stop <- w513 stop-if-true
                    n249 = call <vilib>:"High Resolution Relative Seconds.vi"() -> ("relative seconds"=w516:dbl)
                    n250 = Subtract(x=w516, y=w515) -> (x-y=w514:dbl)
                    n251 = control-ref of="status"() -> (w504:refnum<vi>)
                    n252 = control-ref of="conn ID"() -> (w505:refnum<vi>)
                    n253 = call "TCP Read (SubVI).vi"("Status in"=w504, "TCP in"=w505, "error in (no error)"=w506) -> ("Drv Array"=w510:u8[], "error out"=w503:errorcluster)  [unwired: 2 in, 9 out]
                    n254 = Greater?(x=1.0, y=w514) -> (0:w512:bool)
                    n255 = Index Array(array=w510, index #1=0 ("index")) -> (element #1=w508:u8, element #2=w509:u8)  [unwired: 1 in]
                    n256 = Join Numbers(hi=w509, lo=w508) -> ((hi.lo)=w502:u16)
                    n257 = Equal?(x=w502, y=w501) -> (x = y?=w500:bool)
                    n258 = Compound Arithmetic op=OR(w500, w512, "DataBSendFlag") -> (w513:bool)
                  }
                  n259 = property on="CheckSumData2" class="DigNum (strict)" props=["Value"](error in=w472) -> (error out=w487:errorcluster)  [unwired: 1 in, 2 out]
                  n260 = property on="DataBSendFlag" class="Bool (strict)"(error in=w487, "Value"=FALSE ("DataB")) -> (error out=w486:errorcluster)  [unwired: 1 in, 1 out]
                  n261 = Equal?(x=w482, y=w471) -> (x = y?=w497:bool)
                }
              }
            }
            "Array 4" <- w426
            "Array 5" <- w425
            "array" <- w422
          }
          frame True {
            n262 = control-ref of="State"() -> (w565:refnum<vi>)
            n263 = property class="DigNum (strict)"(reference=w565, error in=w561, "Value"=3) -> (error out=w562:errorcluster)  [unwired: 1 out]
            n264 = flat-sequence {
              tunnel: w562 -> [w629]
              tunnel: [w631] -> w570
              tunnel: [w628] -> w566
              tunnel: w578 -> [w630]
              tunnel: [w629] -> w569
              tunnel: [w628] -> w574
              tunnel: [w628] -> w553
              frame #0 {
                n265 = for {
                  tunnel: w630 -> [w644] mode=indexing
                  shift-right: [w639] -> w631
                  shift-left: u8[] [] -> [w638]
                  shift-right: [w636] -> w628
                  shift-left: u16 0 -> [w637]
                  i -> [w643]
                  n266 = Split Number(x=w644) -> (hi(x)=w635:u8, lo(x)=w634:u8)
                  n267 = Build Array(w635, w634) -> (w641:u8[])
                  n268 = Compound Arithmetic op=ADD(w637, w635, w634) -> (w636:u16)
                  n269 = Multiply(x=w643, y=2) -> (x*y=w640:i32)
                  n270 = Insert Into Array(array=w638, index=w640, new element=w641) -> (w639:u8[])
                }
                "CheckSum Data" <- w628
              }
            }
            n271 = Build Array(w574) -> (w573:u16[])
            n272 = while {
              tunnel: w569 -> [w595]
              tunnel: [w584] -> w563
              shift-right: [w582] -> _
              shift-left: w570 -> [w594]
              tunnel: w568 -> [w588]
              tunnel: w567 -> [w586]
              tunnel: [w581] -> w560
              tunnel: [w580] -> w554 mode=indexing
              i -> [w581]
              stop <- w591 stop-if-true
              n273 = Delete From Array(array=w594, length=24, index=0) -> (deleted portion=w580:u8[], array with subset deleted=w582:u8[])
              n274 = Array Size(array=w582) -> (size(s)=w590:i32)
              n275 = Byte Array To String(unsigned byte array=w580) -> (string=w587:string)
              n276 = Less Or Equal?(x=w590, y=0) -> (x <= y?=w591:bool)
              "Data1Send" <- w591
              n277 = call "TCPSend (SubVI).vi"("Opcode"=u32 4096, "error in"=w595, "string"=w587, "Drv"=w586, "RefNum in"=w588) -> ("error out"=w585:errorcluster)  [unwired: 6 in]
              n278 = flat-sequence {
                tunnel: w585 -> [w596]
                tunnel: [w596] -> w584
                frame #0 {
                  n279 = Wait (ms)(milliseconds to wait=u32 10) -> ()  [unwired: 1 out]
                }
              }
              "Numeric" <- w581
            }
            "Array 2" <- w554
            n280 = feedback #2() -> (w555:i32[])  [unwired: 1 in]
            n281 = Insert Into Array(array=w555, index=w559, new element=w560) -> (w558:i32[])
            "O" <- w558
            n282 = Build Array (concatenate)(w557, w558) -> (w556:i32[])
            n283 = feedback-in #2(w556) -> ()
            n284 = case shown="False" w572 {
              tunnel: w563 -> [w606 w627]
              tunnel: [w602 w627] -> w579
              tunnel: [w599 u16 0 ("Value")] -> w577
              tunnel: [w604 FALSE] -> w571
              tunnel: w553 -> [w598 _]
              frame False {
                n285 = call <vilib>:"High Resolution Relative Seconds.vi"() -> ("relative seconds"=w600:dbl)
                n286 = while {
                  tunnel: w606 -> [w615]
                  tunnel: [w609] -> w605
                  tunnel: ["Data1SendFlag"] -> w604
                  tunnel: w600 -> [w618]
                  tunnel: [w608] -> w599
                  tunnel: w598 -> [w607]
                  stop <- w623 stop-if-true
                  n287 = control-ref of="status"() -> (w616:refnum<vi>)
                  n288 = control-ref of="conn ID"() -> (w617:refnum<vi>)
                  n289 = call <vilib>:"High Resolution Relative Seconds.vi"() -> ("relative seconds"=w619:dbl)
                  n290 = call "TCP Read (SubVI).vi"("Status in"=w616, "TCP in"=w617, "error in (no error)"=w615) -> ("Drv Array"=w613:u8[], "error out"=w609:errorcluster)  [unwired: 2 in, 9 out]
                  n291 = Subtract(x=w619, y=w618) -> (x-y=w620:dbl)
                  n292 = Index Array(array=w613, index #1=0 ("index")) -> (element #1=w611:u8, element #2=w612:u8)  [unwired: 1 in]
                  n293 = Greater?(x=w620, y=1.0) -> (0:w622:bool)
                  n294 = Join Numbers(hi=w612, lo=w611) -> ((hi.lo)=w608:u16)
                  n295 = Equal?(x=w607, y=w608) -> (x = y?=w610:bool)
                  n296 = Compound Arithmetic op=OR(w610, w622, "Data1SendFlag") -> (w623:bool)
                }
                n297 = property on="CheckSumData1" class="DigNum (strict)" props=["Value"](error in=w605) -> (error out=w603:errorcluster)  [unwired: 1 in, 2 out]
                n298 = property on="Data1SendFlag" class="Bool (strict)"(error in=w603, "Value"=FALSE ("Data1")) -> (error out=w602:errorcluster)  [unwired: 1 in, 1 out]
              }
              frame True {
              }
            }
            n299 = Equal?(x=w566, y=w577) -> (x = y?=w576:bool)
            n300 = Build Array(w576) -> (w575:bool[])
          }
        }
      }
      "Array 3" <- w384
      "CheckSum" <- w382
      "CheckSumArray" <- w381
      n301 = Unbundle(w379) -> ("status"=w378:bool)  [unwired: 2 out]
      n302 = Not(x=w378) -> (.not. x?=→"Status":bool)
    }
  }
  n303 = disable-structure shown="Enabled" {
    frame Disabled {
      n304 = call <vilib>:"Application Directory.vi"() -> ("Application Directory"=w657:path)
      n305 = Build Path(base path=w657, name or relative path="ans.txt") -> (appended path=w656:path)
      n306 = Open/Create/Replace File(file path (use dialog)=w656, operation (0:open)=T1."open or create") -> (refnum out=w653:refnum<file>, error out=w654:errorcluster)  [unwired: 4 in, 1 out]
      n307 = for {
        tunnel: _ -> [w669] mode=indexing
        tunnel: w654 -> [w667]
        tunnel: w653 -> [w666]
        i -> [w662]
        n308 = Quotient & Remainder(x=w662, y=24 ("x")) -> (x-y*floor(x/y)=w660:i32)  [unwired: 1 out]
        n309 = Format Into String(format string="%02x", w669) -> (resulting string=w665:string)  [unwired: 2 in, 1 out]
        n310 = Equal?(x=w660, y=0) -> (x = y?=w663:bool)
        n311 = case shown="True" w663 {
          tunnel: w665 -> [w672 w675]
          tunnel: [w671 w674] -> w664
          frame False {
            n312 = call <vilib>:"Space Constant.vi"() -> ("String"=w670:string)
            n313 = Concatenate Strings(w672, w670) -> (w671:string)
          }
          frame True {
            n314 = Concatenate Strings(w675, "\r\n") -> (w674:string)
          }
        }
        n315 = Write to Text File(file (use dialog)=w666, text=w664, error in=w667) -> ()  [unwired: 1 in, 3 out]
      }
    }
    frame Enabled {
    }
  }
  n316 = flat-sequence {
    tunnel: w14 -> [w690]
    tunnel: [w690] -> w7
    tunnel: w9 -> [w689]
    tunnel: w8 -> [w688]
    tunnel: w24 -> [w687]
    frame #0 {
      n317 = Build Array(w689, w688, w687) -> (w682:bool[])
      n318 = for {
        tunnel: w682 -> [w699] mode=indexing
        shift-right: [w697] -> w685
        shift-left: "" -> [w698]
        i -> [w695]
        n319 = case shown="2" w695 {
          tunnel: ["- Autobaud" "- Header Checksum" "- Data Checksum"] -> w692
          frame 0, Default {
          }
          frame 1 {
          }
          frame 2 {
          }
        }
        n320 = Select(t=" Failed !", s=w699, f=" Success !") -> (s? t:f=w691:string)
        n321 = Concatenate Strings(w698, w692, w691, "\r\n") -> (w697:string)
      }
      n322 = Search 1D Array(1D array=w682, element=TRUE) -> (index of element=w680:i32)  [unwired: 1 in]
      n323 = Greater Than 0?(x=w680) -> (x > 0?=w679:bool)
      n324 = Select(t="Try to reset the UUT" ("string"), s=w679, f="Burn Successed.") -> (s? t:f=w677:string)
      n325 = Concatenate Strings(w685, "\r\n", w677) -> (→"Error List":string)
    }
  }
  n326 = control-ref of="conn ID"() -> (w4:refnum<vi>)
  n327 = flat-sequence {
    tunnel: w7 -> [w723]
    tunnel: w23 -> [w722]
    tunnel: w4 -> [w721]
    tunnel: [w703] -> w6
    frame #0 {
      n328 = Split Number(x=u32 0) -> (hi(x)=w716:u16, lo(x)=w715:u16)
      n329 = Split Number(x=w715) -> (hi(x)=w710:u8, lo(x)=w709:u8)
      n330 = Split Number(x=w716) -> (hi(x)=w708:u8, lo(x)=w707:u8)
      n331 = Replace Array Subset(array=u8[] [0, 0, 0, 0, 0, 0, 0, 0] ("unsigned byte array"), new element #1=w709, index #1=0 ("index"), new element #2=w710, new element #3=w707, new element #4=w708) -> (w711:u8[])  [unwired: 3 in]
      n332 = Byte Array To String(unsigned byte array=w711) -> (string=w705:string)
      n333 = call "TCPSend (SubVI).vi"("Opcode"=u32 4112, "error in"=w723, "string"=w705, "Drv"=w722, "RefNum in"=w721) -> ("error out"=w718:errorcluster)  [unwired: 6 in]
      n334 = control-ref of="State"() -> (w720:refnum<vi>)
      n335 = property class="DigNum (strict)"(reference=w720, error in=w718, "Value"=10) -> (error out=w717:errorcluster)  [unwired: 1 out]
      n336 = property on="stop Listen" class="Bool (strict)"(error in=w717, "Value"=TRUE ("stop Listen")) -> (error out=w703:errorcluster)  [unwired: 1 in, 1 out]
    }
  }
  "error out" <- w6
